vi "Comparison.vi"(6 "Y2":sgl, 9 "Length 2":dbl, 10 "Length":dbl, 11 "Y1":sgl) -> (2 "Output":sgl)   [LabVIEW 2012]
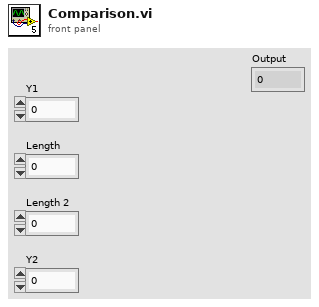
[diagram p1: front panel]
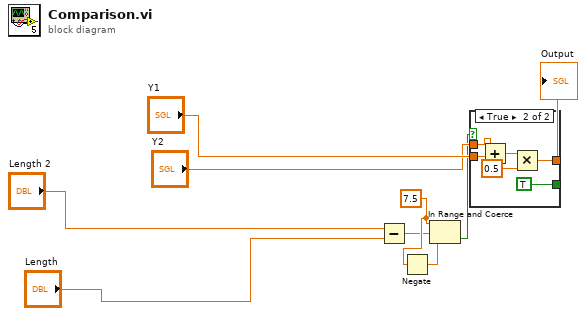
[diagram p0: block diagram]
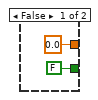
[diagram p2: hidden frame]
diagram:
  w4 = 7.5 ("upper limit")
  n1 = Subtract(x="Length 2", y="Length") -> (x-y=w2:dbl)
  n2 = Negate(x=w4) -> (-x=w5:dbl)
  n3 = In Range and Coerce(upper limit=w4, x=w2, lower limit=w5) -> (In Range?=w3:bool)  [unwired: 1 out]
  n4 = case shown="True" w3 {
    tunnel: "Y2" -> [_ w16]
    tunnel: "Y1" -> [_ w15]
    tunnel: [FALSE TRUE] -> _
    tunnel: [sgl 0.0 w12] -> w1
    frame False {
    }
    frame True {
      n5 = Add(x=w16, y=w15) -> (x+y=w17:sgl)
      n6 = Multiply(x=w17, y=sgl 0.5) -> (x*y=w12:sgl)
    }
  }
  "Output" <- w1
